vi "Close Device.vi"(8 "error in (no error)":errorcluster, 11 "Simulated in":refnum<class "Simulated.lvclass">) -> (0 "error out":errorcluster, 3 "Simulated out":refnum<class "Simulated.lvclass">)   [LabVIEW 2019, in "Simulated.lvclass"]
uses:
  Simulated.lvclass
  Abstract Spectrometer_class/Abstract Spectrometer.lvclass
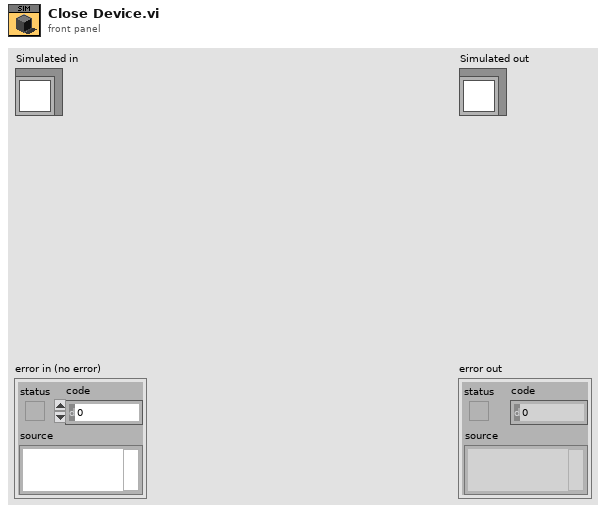
[diagram p1: front panel]
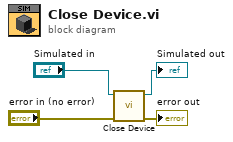
[diagram p0: block diagram]
diagram:
  n1 = call-parent "Close Device.vi"("error in (no error)"="error in (no error)", "Abstract Spectrometer in"="Simulated in") -> ("error out"=→"error out":errorcluster, "Abstract Spectrometer out"=→"Simulated out":refnum<class "Simulated.lvclass">)  [unwired: 8 in]
